vi "Lab Panel V4.86.vi"() -> ()   [LabVIEW 2013] (continued)
                    n882 = stacked-sequence {
                      seq-local: [w1543 _ _ _ _] -> [_ w1567 _ _ _]
                      tunnel: w1542 -> [w1548 _ _ _ _]
                      tunnel: w1541 -> [w1544 _ _ _ _]
                      tunnel: w1540 -> [w1558 _ _ _ _]
                      tunnel: w1539 -> [w1551 _ _ _ _]
                      tunnel: w1538 -> [w1546 _ _ _ _]
                      tunnel: [_ w1562 _ _ _] -> w1537
                      tunnel: w1536 -> [_ _ _ w1587 _]
                      tunnel: w1535 -> [_ _ _ w1586 _]
                      tunnel: w1534 -> [_ _ _ w1585 _]
                      frame #0 {
                        w1545 = "\\"
                        n883 = local read "SET LAB05-1"() -> (w1553:T5)
                        n884 = case shown="\"CYCLE TEST\"" w1558 {
                          tunnel: ["L05-1-CHART TEST-" "L05-1-CYCLE TEST-" "L05-1-T-RISE TEST-"] -> w1554
                          frame "CHART TEST", Default {
                          }
                          frame "CYCLE TEST" {
                          }
                          frame "T-RISE TEST" {
                          }
                        }
                        n885 = Unbundle(w1553) -> ("DESCRIPTION"=w1552:string)  [unwired: 4 out]
                        n886 = Concatenate Strings(w1548, "\\", w1546, w1545, w1544, w1545) -> (w1555:string)
                        n887 = String To Path(string=w1555) -> (path=w1557:path)
                        n888 = Concatenate Strings(w1555, w1554, w1552, "-", w1551, ".tdms") -> (w1543:string)
                        n889 = Create Folder(path (use dialog)=w1557) -> (error out=w1556:errorcluster)  [unwired: 2 in, 2 out]
                        n890 = global write "Global 1.vi" "LAB05-1 FILE"(w1543) -> ()
                        n891 = call <vilib>:"Clear Errors.vi"("error in (no error)"=w1556) -> ()  [unwired: 6 in, 1 out]
                      }
                      frame #1 {
                        (unwired) FALSE
                        n892 = String To Path(string=w1567) -> (path=w1563:path)
                        n893 = TDMS Open(6:FALSE, 10:T18."create or replace" ("operation (0:open)"), 11:w1563) -> (0:w1562:errorcluster, 3:→"TDMS LAB05-1":refnum<k34>)  [unwired: 4 in]
                      }
                      frame #2 {
                        n894 = local read "SET LAB05-1"() -> (w1573:T5)
                        n895 = local read "TDMS LAB05-1"() -> (w1584:refnum<k34>)
                        n896 = Build Array("Testers Name", "Description", "Set Test Cycles", "T-Rise minutes", "T-Rise Deg C") -> (w1574:string[])
                        n897 = Unbundle(w1573) -> ("NAME"=w1572:string, "DESCRIPTION"=w1571:string, "CYCLES"=w1570:dbl, "T-RISE mins"=w1569:dbl, "T-RISE deg C"=w1568:dbl)
                        n898 = Number To Decimal String(number=w1570) -> (decimal integer string=w1583:string)  [unwired: 1 in]
                        n899 = Number To Decimal String(number=w1569) -> (decimal integer string=w1582:string)  [unwired: 1 in]
                        n900 = Number To Decimal String(number=w1568) -> (decimal integer string=w1581:string)  [unwired: 1 in]
                        n901 = Build Array(w1572, w1571, w1583, w1582, w1581) -> (w1580:string[])
                        n902 = TDMS Set Properties(5:w1580, 7:w1574, 11:w1584) -> ()  [unwired: 3 in, 4 out]
                      }
                      frame #3 {
                        n903 = local read "DISP LAB05-1"() -> (w1589:T4)
                        n904 = Concatenate Strings("LAB05-1  ", w1587) -> (w1590:string)
                        n905 = Two Button Dialog(message=w1590, 1:w1585, 2:w1586) -> (T button?=w1592:bool)
                        n906 = case shown="True" w1592 {
                          tunnel: w1589 -> [w1599 w1600]
                          tunnel: [w1599 w1600] -> w1596
                          tunnel: [w1598 w1601] -> w1595
                          tunnel: [w1597 w1601] -> w1594
                          frame False {
                            n907 = Unbundle(w1599) -> ("CYCLE"=w1598:dbl, "MINS"=w1597:dbl)  [unwired: 1 out]
                          }
                          frame True {
                            w1601 = 0.0
                          }
                        }
                        n908 = Bundle(cluster=w1596, "CYCLE"=w1595, "MINS"=w1594, "STATUS"="RUN") -> (w1588:T4)
                        n909 = local write "DISP LAB05-1"(w1588) -> ()
                      }
                      frame #4 {
                        n910 = local read "SIG LAB05-1"() -> (w1604:T2)
                        n911 = local read "TEMP START LAB05-1"() -> (w1606:cluster{"TL":dbl, "TN":dbl})
                        n912 = Unbundle(w1604) -> ("Tmp Live"=w1603:dbl, "Tmp Neut"=w1602:dbl)  [unwired: 3 out]
                        n913 = Bundle(cluster=w1606, "TL"=w1603, "TN"=w1602) -> (w1605:cluster{"TL":dbl, "TN":dbl})
                        n914 = local write "TEMP START LAB05-1"(w1605) -> ()
                      }
                    }
                  }
                }
              }
              event "RUN LAB05-2": Value Change {
                n915 = event-data() -> ("NewVal"=w1610:bool)  [unwired: 1 in, 5 out]
                n916 = local write "run lab05-2"(w1610) -> ()
                n917 = case shown="True" w1610 {
                  tunnel: w1616 -> [_ w1652]
                  tunnel: w1615 -> [_ w1651]
                  tunnel: w1613 -> [w1618 w1650]
                  tunnel: w1614 -> [_ w1649]
                  tunnel: w1612 -> [_ w1648]
                  tunnel: [w1617 w1647] -> w1611
                  tunnel: w1609 -> [_ w1646]
                  tunnel: w1608 -> [_ w1645]
                  tunnel: w1607 -> [_ w1644]
                  frame False {
                    # "stop test"
                    n918 = stacked-sequence {
                      tunnel: w1618 -> [w1627 _]
                      tunnel: [w1619 _] -> w1617
                      frame #0 {
                        n919 = local read "DISP LAB05-2"() -> (w1626:T4)
                        n920 = Unbundle(w1626) -> ("CYCLE"=w1624:dbl, "MINS"=w1625:dbl)  [unwired: 1 out]
                        n921 = case shown="\"CYCLE TEST\"" w1627 {
                          tunnel: w1625 -> [_ _ w1634]
                          tunnel: w1624 -> [w1632 w1633 _]
                          tunnel: [w1632 w1633 w1634] -> w1623
                          frame "CHART TEST", Default {
                          }
                          frame "CYCLE TEST" {
                          }
                          frame "T-RISE TEST" {
                          }
                        }
                        n922 = local read "TDMS LAB05-2"() -> (w1631:refnum<k34>)
                        n923 = Build Array("STOPPED") -> (w1628:string[])
                        n924 = Build Array(w1623) -> (w1622:dbl[])
                        n925 = TDMS Write(0:w1631, 5:"TEST RESULT", 7:w1628, 9:w1622) -> (4:w1620:refnum<k34>, 15:w1621:errorcluster)  [unwired: 2 in, 2 out]
                        n926 = TDMS Close(8:w1621, 11:w1620) -> (0:w1619:errorcluster)  [unwired: 1 out]
                      }
                      frame #1 {
                        n927 = local read "DISP LAB05-2"() -> (w1638:T4)
                        n928 = stacked-sequence {
                          tunnel: "LAB05-2" -> [w1640 w1642]
                          frame #0 {
                            n929 = call "sub vi - defrag tdms v1.vi"("panel id"=w1640) -> ("error out"=w1639:errorcluster)  [unwired: 10 in]
                            n930 = local write "data file error"(w1639) -> ()
                          }
                          frame #1 {
                            n931 = local write "RESULT LAB05-2"(FALSE) -> ()
                            n932 = call "Save data file to network drive v2.vi"("panel id"=w1642) -> ("network file save error"=w1641:errorcluster)  [unwired: 9 in, 1 out]
                            n933 = local write "data file error"(w1641) -> ()
                          }
                        }
                        n934 = Bundle(cluster=w1638, "STATUS"="STOP") -> (w1636:T4)  [unwired: 2 in]
                        n935 = local write "DISP LAB05-2"(w1636) -> ()
                      }
                    }
                  }
                  frame True {
                    # "start new test and create test file"
                    n936 = stacked-sequence {
                      seq-local: [w1653 _ _ _ _] -> [_ w1677 _ _ _]
                      tunnel: w1652 -> [w1658 _ _ _ _]
                      tunnel: w1651 -> [w1654 _ _ _ _]
                      tunnel: w1650 -> [w1668 _ _ _ _]
                      tunnel: w1649 -> [w1661 _ _ _ _]
                      tunnel: w1648 -> [w1656 _ _ _ _]
                      tunnel: [_ w1672 _ _ _] -> w1647
                      tunnel: w1646 -> [_ _ _ w1697 _]
                      tunnel: w1645 -> [_ _ _ w1696 _]
                      tunnel: w1644 -> [_ _ _ w1695 _]
                      frame #0 {
                        w1655 = "\\"
                        n937 = local read "SET LAB05-2"() -> (w1663:T5)
                        n938 = case shown="\"CYCLE TEST\"" w1668 {
                          tunnel: ["L05-2-CHART TEST-" "L05-2-CYCLE TEST-" "L05-2-T-RISE TEST-"] -> w1664
                          frame "CHART TEST", Default {
                          }
                          frame "CYCLE TEST" {
                          }
                          frame "T-RISE TEST" {
                          }
                        }
                        n939 = Unbundle(w1663) -> ("DESCRIPTION"=w1662:string)  [unwired: 4 out]
                        n940 = Concatenate Strings(w1658, "\\", w1656, w1655, w1654, w1655) -> (w1665:string)
                        n941 = String To Path(string=w1665) -> (path=w1667:path)
                        n942 = Concatenate Strings(w1665, w1664, w1662, "-", w1661, ".tdms") -> (w1653:string)
                        n943 = Create Folder(path (use dialog)=w1667) -> (error out=w1666:errorcluster)  [unwired: 2 in, 2 out]
                        n944 = global write "Global 1.vi" "LAB05-2 FILE"(w1653) -> ()
                        n945 = call <vilib>:"Clear Errors.vi"("error in (no error)"=w1666) -> ()  [unwired: 6 in, 1 out]
                      }
                      frame #1 {
                        (unwired) FALSE
                        n946 = String To Path(string=w1677) -> (path=w1673:path)
                        n947 = TDMS Open(6:FALSE, 10:T18."create or replace" ("operation (0:open)"), 11:w1673) -> (0:w1672:errorcluster, 3:→"TDMS LAB05-2":refnum<k34>)  [unwired: 4 in]
                      }
                      frame #2 {
                        n948 = local read "SET LAB05-2"() -> (w1683:T5)
                        n949 = local read "TDMS LAB05-2"() -> (w1694:refnum<k34>)
                        n950 = Build Array("Testers Name", "Description", "Set Test Cycles", "T-Rise minutes", "T-Rise Deg C") -> (w1684:string[])
                        n951 = Unbundle(w1683) -> ("NAME"=w1682:string, "DESCRIPTION"=w1681:string, "CYCLES"=w1680:dbl, "T-RISE mins"=w1679:dbl, "T-RISE deg C"=w1678:dbl)
                        n952 = Number To Decimal String(number=w1680) -> (decimal integer string=w1693:string)  [unwired: 1 in]
                        n953 = Number To Decimal String(number=w1679) -> (decimal integer string=w1692:string)  [unwired: 1 in]
                        n954 = Number To Decimal String(number=w1678) -> (decimal integer string=w1691:string)  [unwired: 1 in]
                        n955 = Build Array(w1682, w1681, w1693, w1692, w1691) -> (w1690:string[])
                        n956 = TDMS Set Properties(5:w1690, 7:w1684, 11:w1694) -> ()  [unwired: 3 in, 4 out]
                      }
                      frame #3 {
                        n957 = local read "DISP LAB05-2"() -> (w1699:T4)
                        n958 = Concatenate Strings("LAB05-2  ", w1697) -> (w1700:string)
                        n959 = Two Button Dialog(message=w1700, 1:w1695, 2:w1696) -> (T button?=w1702:bool)
                        n960 = case shown="True" w1702 {
                          tunnel: w1699 -> [w1709 w1710]
                          tunnel: [w1709 w1710] -> w1706
                          tunnel: [w1708 w1711] -> w1705
                          tunnel: [w1707 w1711] -> w1704
                          frame False {
                            n961 = Unbundle(w1709) -> ("CYCLE"=w1708:dbl, "MINS"=w1707:dbl)  [unwired: 1 out]
                          }
                          frame True {
                            w1711 = 0.0
                          }
                        }
                        n962 = Bundle(cluster=w1706, "CYCLE"=w1705, "MINS"=w1704, "STATUS"="RUN") -> (w1698:T4)
                        n963 = local write "DISP LAB05-2"(w1698) -> ()
                      }
                      frame #4 {
                        n964 = local read "SIG LAB05-2"() -> (w1714:T2)
                        n965 = local read "TEMP START LAB05-2"() -> (w1716:cluster{"TL":dbl, "TN":dbl})
                        n966 = Unbundle(w1714) -> ("Tmp Live"=w1713:dbl, "Tmp Neut"=w1712:dbl)  [unwired: 3 out]
                        n967 = Bundle(cluster=w1716, "TL"=w1713, "TN"=w1712) -> (w1715:cluster{"TL":dbl, "TN":dbl})
                        n968 = local write "TEMP START LAB05-2"(w1715) -> ()
                      }
                    }
                  }
                }
              }
            }
            n969 = local write "data file error"(w588) -> ()
          }
          frame #4 {
            # "check if test cycles reached for cycle tests, if so then test pass"
            n970 = stacked-sequence {
              tunnel: w1736 -> [_ _ _ _ _ _ _ _ _ _]
              tunnel: w1735 -> [_ _ _ _ _ _ _ _ _ _]
              tunnel: w1734 -> [_ _ _ _ _ _ _ _ _ _]
              tunnel: w1733 -> [_ _ _ _ _ _ _ _ _ _]
              tunnel: w1732 -> [_ _ _ _ _ _ _ _ _ _]
              tunnel: w1731 -> [_ _ _ _ _ _ _ _ _ _]
              tunnel: w1730 -> [_ _ _ _ _ _ _ _ _ _]
              tunnel: w1729 -> [_ _ _ _ _ _ _ _ _ _]
              tunnel: w1728 -> [_ _ _ _ _ _ _ _ _ _]
              tunnel: w1727 -> [_ _ _ _ _ _ _ _ _ _]
              tunnel: w1726 -> [w1742 _ _ _ _ _ _ _ _ _]
              tunnel: w1725 -> [_ w1777 _ _ _ _ _ _ _ _]
              tunnel: w1724 -> [_ _ w1817 _ _ _ _ _ _ _]
              tunnel: w1723 -> [_ _ _ w1857 _ _ _ _ _ _]
              tunnel: w1722 -> [_ _ _ _ w1897 _ _ _ _ _]
              tunnel: w1721 -> [_ _ _ _ _ w1937 _ _ _ _]
              tunnel: w1720 -> [_ _ _ _ _ _ w1977 _ _ _]
              tunnel: w1719 -> [_ _ _ _ _ _ _ w2017 _ _]
              tunnel: w1718 -> [_ _ _ _ _ _ _ _ w2057 _]
              tunnel: w1717 -> [_ _ _ _ _ _ _ _ _ w2097]
              frame #0 {
                # "LAB01-1"
                n971 = Less?(x=w1742, y=2) -> (x < y?=w1740:bool)
                n972 = local read "DISP LAB01-1"() -> (w1743:T4)
                n973 = Unbundle(w1743) -> ("STATUS"=w1737:string)  [unwired: 2 out]
                n974 = Equal?(x=w1737, y="RUN") -> (x = y?=w1739:bool)
                n975 = And(x=w1739, y=w1740) -> (x .and. y?=w1738:bool)
                n976 = case shown="True" w1738 {
                  tunnel: w1743 -> [_ w1748]
                  tunnel: w1742 -> [_ w1752]
                  frame False {
                  }
                  frame True {
                    n977 = local read "SET LAB01-1"() -> (w1754:T5)
                    n978 = local read "TDMS LAB01-1"() -> (w1747:refnum<k34>)
                    n979 = Unbundle(w1754) -> ("CYCLES"=w1745:dbl, "T-RISE mins"=w1751:dbl)  [unwired: 3 out]
                    n980 = case shown="\"CYCLE TEST\"" w1752 {
                      tunnel: w1751 -> [_ _ w1761]
                      tunnel: [w1756 w1758 w1761] -> w1750
                      tunnel: w1745 -> [w1756 w1758 _]
                      tunnel: ["CHART PASS" "CYCLE PASS" "T-RISE PASS"] -> w1749
                      frame "CHART TEST", Default {
                      }
                      frame "CYCLE TEST" {
                      }
                      frame "T-RISE TEST" {
                      }
                    }
                    n981 = Unbundle(w1748) -> ("CYCLE"=w1753:dbl)  [unwired: 2 out]
                    n982 = Increment(x=w1745) -> (x+1=w1746:dbl)
                    n983 = Greater Or Equal?(x=w1753, y=w1746) -> (x >= y?=w1755:bool)
                    n984 = case shown="True" w1755 {
                      tunnel: w1750 -> [w1765 _]
                      tunnel: w1749 -> [w1764 _]
                      tunnel: w1748 -> [w1763 _]
                      tunnel: w1747 -> [w1762 _]
                      frame True {
                        n985 = stacked-sequence {
                          tunnel: w1765 -> [w1769 _]
                          tunnel: w1764 -> [w1767 w1773]
                          tunnel: w1763 -> [_ w1776]
                          tunnel: w1762 -> [w1766 _]
                          frame #0 {
                            n986 = Build Array(w1767) -> (w1770:string[])
                            n987 = Build Array(w1769) -> (w1768:dbl[])
                            n988 = TDMS Write(0:w1766, 5:"TEST PASS", 7:w1770, 9:w1768) -> (15:w1772:errorcluster)  [unwired: 2 in, 3 out]
                            n989 = local write "data file error"(w1772) -> ()
                          }
                          frame #1 {
                            n990 = Bundle(cluster=w1776, "STATUS"=w1773) -> (w1774:T4)  [unwired: 2 in]
                            n991 = local write "RESULT LAB01-1"(TRUE) -> ()
                            n992 = local write "DISP LAB01-1"(w1774) -> ()
                          }
                        }
                      }
                      frame False {
                      }
                    }
                  }
                }
              }
              frame #1 {
                # "LAB01-2"
                n993 = Less?(x=w1777, y=2) -> (x < y?=w1780:bool)
                n994 = local read "DISP LAB01-2"() -> (w1782:T4)
                n995 = Unbundle(w1782) -> ("STATUS"=w1783:string)  [unwired: 2 out]
                n996 = Equal?(x=w1783, y="RUN") -> (x = y?=w1779:bool)
                n997 = And(x=w1779, y=w1780) -> (x .and. y?=w1778:bool)
                n998 = case shown="True" w1778 {
                  tunnel: w1782 -> [_ w1788]
                  tunnel: w1777 -> [_ w1792]
                  frame False {
                  }
                  frame True {
                    n999 = local read "SET LAB01-2"() -> (w1794:T5)
                    n1000 = local read "TDMS LAB01-2"() -> (w1787:refnum<k34>)
                    n1001 = Unbundle(w1794) -> ("CYCLES"=w1785:dbl, "T-RISE mins"=w1791:dbl)  [unwired: 3 out]
                    n1002 = case shown="\"T-RISE TEST\"" w1792 {
                      tunnel: w1791 -> [_ _ w1801]
                      tunnel: [w1796 w1798 w1801] -> w1790
                      tunnel: w1785 -> [w1796 w1798 _]
                      tunnel: ["CHART PASS" "CYCLE PASS" "T-RISE PASS"] -> w1789
                      frame "CHART TEST", Default {
                      }
                      frame "CYCLE TEST" {
                      }
                      frame "T-RISE TEST" {
                      }
                    }
                    n1003 = Unbundle(w1788) -> ("CYCLE"=w1793:dbl)  [unwired: 2 out]
                    n1004 = Increment(x=w1785) -> (x+1=w1786:dbl)
                    n1005 = Greater Or Equal?(x=w1793, y=w1786) -> (x >= y?=w1795:bool)
                    n1006 = case shown="True" w1795 {
                      tunnel: w1790 -> [w1805 _]
                      tunnel: w1789 -> [w1804 _]
                      tunnel: w1788 -> [w1803 _]
                      tunnel: w1787 -> [w1802 _]
                      frame True {
                        n1007 = stacked-sequence {
                          tunnel: w1805 -> [w1809 _]
                          tunnel: w1804 -> [w1807 w1813]
                          tunnel: w1803 -> [_ w1816]
                          tunnel: w1802 -> [w1806 _]
                          frame #0 {
                            n1008 = Build Array(w1807) -> (w1810:string[])
                            n1009 = Build Array(w1809) -> (w1808:dbl[])
                            n1010 = TDMS Write(0:w1806, 5:"TEST PASS", 7:w1810, 9:w1808) -> (15:w1812:errorcluster)  [unwired: 2 in, 3 out]
                            n1011 = local write "data file error"(w1812) -> ()
                          }
                          frame #1 {
                            n1012 = Bundle(cluster=w1816, "STATUS"=w1813) -> (w1814:T4)  [unwired: 2 in]
                            n1013 = local write "RESULT LAB01-2"(TRUE) -> ()
                            n1014 = local write "DISP LAB01-2"(w1814) -> ()
                          }
                        }
                      }
                      frame False {
                      }
                    }
                  }
                }
              }
              frame #2 {
                # "LAB02-1"
                n1015 = Less?(x=w1817, y=2) -> (x < y?=w1820:bool)
                n1016 = local read "DISP LAB02-1"() -> (w1822:T4)
                n1017 = Unbundle(w1822) -> ("STATUS"=w1823:string)  [unwired: 2 out]
                n1018 = Equal?(x=w1823, y="RUN") -> (x = y?=w1819:bool)
                n1019 = And(x=w1819, y=w1820) -> (x .and. y?=w1818:bool)
                n1020 = case shown="True" w1818 {
                  tunnel: w1822 -> [_ w1828]
                  tunnel: w1817 -> [_ w1832]
                  frame False {
                  }
                  frame True {
                    n1021 = local read "SET LAB02-1"() -> (w1834:T5)
                    n1022 = local read "TDMS LAB02-1"() -> (w1827:refnum<k34>)
                    n1023 = Unbundle(w1828) -> ("CYCLE"=w1833:dbl)  [unwired: 2 out]
                    n1024 = Unbundle(w1834) -> ("CYCLES"=w1825:dbl, "T-RISE mins"=w1831:dbl)  [unwired: 3 out]
                    n1025 = case shown="\"T-RISE TEST\"" w1832 {
                      tunnel: w1831 -> [_ _ w1841]
                      tunnel: [w1836 w1838 w1841] -> w1830
                      tunnel: w1825 -> [w1836 w1838 _]
                      tunnel: ["CHART PASS" "CYCLE PASS" "T-RISE PASS"] -> w1829
                      frame "CHART TEST", Default {
                      }
                      frame "CYCLE TEST" {
                      }
                      frame "T-RISE TEST" {
                      }
                    }
                    n1026 = Increment(x=w1825) -> (x+1=w1826:dbl)
                    n1027 = Greater Or Equal?(x=w1833, y=w1826) -> (x >= y?=w1835:bool)
                    n1028 = case shown="True" w1835 {
                      tunnel: w1830 -> [w1845 _]
                      tunnel: w1829 -> [w1844 _]
                      tunnel: w1828 -> [w1843 _]
                      tunnel: w1827 -> [w1842 _]
                      frame True {
                        n1029 = stacked-sequence {
                          tunnel: w1845 -> [w1849 _]
                          tunnel: w1844 -> [w1847 w1853]
                          tunnel: w1843 -> [_ w1856]
                          tunnel: w1842 -> [w1846 _]
                          frame #0 {
                            n1030 = Build Array(w1847) -> (w1850:string[])
                            n1031 = Build Array(w1849) -> (w1848:dbl[])
                            n1032 = TDMS Write(0:w1846, 5:"TEST PASS", 7:w1850, 9:w1848) -> (15:w1852:errorcluster)  [unwired: 2 in, 3 out]
                            n1033 = local write "data file error"(w1852) -> ()
                          }
                          frame #1 {
                            n1034 = Bundle(cluster=w1856, "STATUS"=w1853) -> (w1854:T4)  [unwired: 2 in]
                            n1035 = local write "RESULT LAB02-1"(TRUE) -> ()
                            n1036 = local write "DISP LAB02-1"(w1854) -> ()
                          }
                        }
                      }
                      frame False {
                      }
                    }
                  }
                }
              }
              frame #3 {
                # "LAB02-2"
                n1037 = Less?(x=w1857, y=2) -> (x < y?=w1860:bool)
                n1038 = local read "DISP LAB02-2"() -> (w1862:T4)
                n1039 = Unbundle(w1862) -> ("STATUS"=w1863:string)  [unwired: 2 out]
                n1040 = Equal?(x=w1863, y="RUN") -> (x = y?=w1859:bool)
                n1041 = And(x=w1859, y=w1860) -> (x .and. y?=w1858:bool)
                n1042 = case shown="True" w1858 {
                  tunnel: w1862 -> [_ w1868]
                  tunnel: w1857 -> [_ w1872]
                  frame False {
                  }
                  frame True {
                    n1043 = local read "SET LAB02-2"() -> (w1874:T5)
                    n1044 = local read "TDMS LAB02-2"() -> (w1867:refnum<k34>)
                    n1045 = Unbundle(w1868) -> ("CYCLE"=w1873:dbl)  [unwired: 2 out]
                    n1046 = Unbundle(w1874) -> ("CYCLES"=w1865:dbl, "T-RISE mins"=w1871:dbl)  [unwired: 3 out]
                    n1047 = case shown="\"T-RISE TEST\"" w1872 {
                      tunnel: w1871 -> [_ _ w1881]
                      tunnel: [w1876 w1878 w1881] -> w1870
                      tunnel: w1865 -> [w1876 w1878 _]
                      tunnel: ["CHART PASS" "CYCLE PASS" "T-RISE PASS"] -> w1869
                      frame "CHART TEST", Default {
                      }
                      frame "CYCLE TEST" {
                      }
                      frame "T-RISE TEST" {
                      }
                    }
                    n1048 = Increment(x=w1865) -> (x+1=w1866:dbl)
                    n1049 = Greater Or Equal?(x=w1873, y=w1866) -> (x >= y?=w1875:bool)
                    n1050 = case shown="True" w1875 {
                      tunnel: w1870 -> [w1885 _]
                      tunnel: w1869 -> [w1884 _]
                      tunnel: w1868 -> [w1883 _]
                      tunnel: w1867 -> [w1882 _]
                      frame True {
                        n1051 = stacked-sequence {
                          tunnel: w1885 -> [w1889 _]
                          tunnel: w1884 -> [w1887 w1893]
                          tunnel: w1883 -> [_ w1896]
                          tunnel: w1882 -> [w1886 _]
                          frame #0 {
                            n1052 = Build Array(w1887) -> (w1890:string[])
                            n1053 = Build Array(w1889) -> (w1888:dbl[])
                            n1054 = TDMS Write(0:w1886, 5:"TEST PASS", 7:w1890, 9:w1888) -> (15:w1892:errorcluster)  [unwired: 2 in, 3 out]
                            n1055 = local write "data file error"(w1892) -> ()
                          }
                          frame #1 {
                            n1056 = Bundle(cluster=w1896, "STATUS"=w1893) -> (w1894:T4)  [unwired: 2 in]
                            n1057 = local write "RESULT LAB02-2"(TRUE) -> ()
                            n1058 = local write "DISP LAB02-2"(w1894) -> ()
                          }
                        }
                      }
                      frame False {
                      }
                    }
                  }
                }
              }
              frame #4 {
                # "LAB03-1"
                n1059 = Less?(x=w1897, y=2) -> (x < y?=w1900:bool)
                n1060 = local read "DISP LAB03-1"() -> (w1902:T4)
                n1061 = Unbundle(w1902) -> ("STATUS"=w1903:string)  [unwired: 2 out]
                n1062 = Equal?(x=w1903, y="RUN") -> (x = y?=w1899:bool)
                n1063 = And(x=w1899, y=w1900) -> (x .and. y?=w1898:bool)
                n1064 = case shown="True" w1898 {
                  tunnel: w1902 -> [_ w1908]
                  tunnel: w1897 -> [_ w1912]
                  frame False {
                  }
                  frame True {
                    n1065 = local read "SET LAB03-1"() -> (w1914:T5)
                    n1066 = local read "TDMS LAB03-1"() -> (w1907:refnum<k34>)
                    n1067 = Unbundle(w1908) -> ("CYCLE"=w1913:dbl)  [unwired: 2 out]
                    n1068 = Unbundle(w1914) -> ("CYCLES"=w1905:dbl, "T-RISE mins"=w1911:dbl)  [unwired: 3 out]
                    n1069 = case shown="\"T-RISE TEST\"" w1912 {
                      tunnel: w1911 -> [_ _ w1921]
                      tunnel: [w1916 w1918 w1921] -> w1910
                      tunnel: w1905 -> [w1916 w1918 _]
                      tunnel: ["CHART PASS" "CYCLE PASS" "T-RISE PASS"] -> w1909
                      frame "CHART TEST", Default {
                      }
                      frame "CYCLE TEST" {
                      }
                      frame "T-RISE TEST" {
                      }
                    }
                    n1070 = Increment(x=w1905) -> (x+1=w1906:dbl)
                    n1071 = Greater Or Equal?(x=w1913, y=w1906) -> (x >= y?=w1915:bool)
                    n1072 = case shown="True" w1915 {
                      tunnel: w1910 -> [w1925 _]
                      tunnel: w1909 -> [w1924 _]
                      tunnel: w1908 -> [w1923 _]
                      tunnel: w1907 -> [w1922 _]
                      frame True {
                        n1073 = stacked-sequence {
                          tunnel: w1925 -> [w1929 _]
                          tunnel: w1924 -> [w1927 w1933]
                          tunnel: w1923 -> [_ w1936]
                          tunnel: w1922 -> [w1926 _]
                          frame #0 {
                            n1074 = Build Array(w1927) -> (w1930:string[])
                            n1075 = Build Array(w1929) -> (w1928:dbl[])
                            n1076 = TDMS Write(0:w1926, 5:"TEST PASS", 7:w1930, 9:w1928) -> (15:w1932:errorcluster)  [unwired: 2 in, 3 out]
                            n1077 = local write "data file error"(w1932) -> ()
                          }
                          frame #1 {
                            n1078 = Bundle(cluster=w1936, "STATUS"=w1933) -> (w1934:T4)  [unwired: 2 in]
                            n1079 = local write "RESULT LAB03-1"(TRUE) -> ()
                            n1080 = local write "DISP LAB03-1"(w1934) -> ()
                          }
                        }
                      }
                      frame False {
                      }
                    }
                  }
                }
              }
              frame #5 {
                # "LAB03-2"
                n1081 = Less?(x=w1937, y=2) -> (x < y?=w1940:bool)
                n1082 = local read "DISP LAB03-2"() -> (w1942:T4)
                n1083 = Unbundle(w1942) -> ("STATUS"=w1943:string)  [unwired: 2 out]
                n1084 = Equal?(x=w1943, y="RUN") -> (x = y?=w1939:bool)
                n1085 = And(x=w1939, y=w1940) -> (x .and. y?=w1938:bool)
                n1086 = case shown="True" w1938 {
                  tunnel: w1942 -> [_ w1948]
                  tunnel: w1937 -> [_ w1952]
                  frame False {
                  }
                  frame True {
                    n1087 = local read "SET LAB03-2"() -> (w1954:T5)
                    n1088 = local read "TDMS LAB03-2"() -> (w1947:refnum<k34>)
                    n1089 = Unbundle(w1948) -> ("CYCLE"=w1953:dbl)  [unwired: 2 out]
                    n1090 = Unbundle(w1954) -> ("CYCLES"=w1945:dbl, "T-RISE mins"=w1951:dbl)  [unwired: 3 out]
                    n1091 = case shown="\"T-RISE TEST\"" w1952 {
                      tunnel: w1951 -> [_ _ w1961]
                      tunnel: [w1956 w1958 w1961] -> w1950
                      tunnel: w1945 -> [w1956 w1958 _]
                      tunnel: ["CHART PASS" "CYCLE PASS" "T-RISE PASS"] -> w1949
                      frame "CHART TEST", Default {
                      }
                      frame "CYCLE TEST" {
                      }
                      frame "T-RISE TEST" {
                      }
                    }
                    n1092 = Increment(x=w1945) -> (x+1=w1946:dbl)
                    n1093 = Greater Or Equal?(x=w1953, y=w1946) -> (x >= y?=w1955:bool)
                    n1094 = case shown="True" w1955 {
                      tunnel: w1950 -> [w1965 _]
                      tunnel: w1949 -> [w1964 _]
                      tunnel: w1948 -> [w1963 _]
                      tunnel: w1947 -> [w1962 _]
                      frame True {
                        n1095 = stacked-sequence {
                          tunnel: w1965 -> [w1969 _]
                          tunnel: w1964 -> [w1967 w1973]
                          tunnel: w1963 -> [_ w1976]
                          tunnel: w1962 -> [w1966 _]
                          frame #0 {
                            n1096 = Build Array(w1967) -> (w1970:string[])
                            n1097 = Build Array(w1969) -> (w1968:dbl[])
                            n1098 = TDMS Write(0:w1966, 5:"TEST PASS", 7:w1970, 9:w1968) -> (15:w1972:errorcluster)  [unwired: 2 in, 3 out]
                            n1099 = local write "data file error"(w1972) -> ()
                          }
                          frame #1 {
                            n1100 = Bundle(cluster=w1976, "STATUS"=w1973) -> (w1974:T4)  [unwired: 2 in]
                            n1101 = local write "RESULT LAB03-2"(TRUE) -> ()
                            n1102 = local write "DISP LAB03-2"(w1974) -> ()
                          }
                        }
                      }
                      frame False {
                      }
                    }
                  }
                }
              }
              frame #6 {
                # "LAB04-1"
                n1103 = Less?(x=w1977, y=2) -> (x < y?=w1980:bool)
                n1104 = local read "DISP LAB04-1"() -> (w1982:T4)
                n1105 = Unbundle(w1982) -> ("STATUS"=w1983:string)  [unwired: 2 out]
                n1106 = Equal?(x=w1983, y="RUN") -> (x = y?=w1979:bool)
                n1107 = And(x=w1979, y=w1980) -> (x .and. y?=w1978:bool)
                n1108 = case shown="True" w1978 {
                  tunnel: w1982 -> [_ w1988]
                  tunnel: w1977 -> [_ w1992]
                  frame False {
                  }
                  frame True {
                    n1109 = local read "SET LAB04-1"() -> (w1994:T5)
                    n1110 = local read "TDMS LAB04-1"() -> (w1987:refnum<k34>)
                    n1111 = Unbundle(w1988) -> ("CYCLE"=w1993:dbl)  [unwired: 2 out]
                    n1112 = Unbundle(w1994) -> ("CYCLES"=w1985:dbl, "T-RISE mins"=w1991:dbl)  [unwired: 3 out]
                    n1113 = case shown="\"T-RISE TEST\"" w1992 {
                      tunnel: w1991 -> [_ _ w2001]
                      tunnel: [w1996 w1998 w2001] -> w1990
                      tunnel: w1985 -> [w1996 w1998 _]
                      tunnel: ["CHART PASS" "CYCLE PASS" "T-RISE PASS"] -> w1989
                      frame "CHART TEST", Default {
                      }
                      frame "CYCLE TEST" {
                      }
                      frame "T-RISE TEST" {
                      }
                    }
                    n1114 = Increment(x=w1985) -> (x+1=w1986:dbl)
                    n1115 = Greater Or Equal?(x=w1993, y=w1986) -> (x >= y?=w1995:bool)
                    n1116 = case shown="True" w1995 {
                      tunnel: w1990 -> [w2005 _]
                      tunnel: w1989 -> [w2004 _]
                      tunnel: w1988 -> [w2003 _]
                      tunnel: w1987 -> [w2002 _]
                      frame True {
                        n1117 = stacked-sequence {
                          tunnel: w2005 -> [w2009 _]
                          tunnel: w2004 -> [w2007 w2013]
                          tunnel: w2003 -> [_ w2016]
                          tunnel: w2002 -> [w2006 _]
                          frame #0 {
                            n1118 = Build Array(w2007) -> (w2010:string[])
                            n1119 = Build Array(w2009) -> (w2008:dbl[])
                            n1120 = TDMS Write(0:w2006, 5:"TEST PASS", 7:w2010, 9:w2008) -> (15:w2012:errorcluster)  [unwired: 2 in, 3 out]
                            n1121 = local write "data file error"(w2012) -> ()
                          }
                          frame #1 {
                            n1122 = Bundle(cluster=w2016, "STATUS"=w2013) -> (w2014:T4)  [unwired: 2 in]
                            n1123 = local write "RESULT LAB04-1"(TRUE) -> ()
                            n1124 = local write "DISP LAB04-1"(w2014) -> ()
                          }
                        }
                      }
                      frame False {
                      }
                    }
                  }
                }
              }
              frame #7 {
                # "LAB04-2"
                n1125 = Less?(x=w2017, y=2) -> (x < y?=w2020:bool)
                n1126 = local read "DISP LAB04-2"() -> (w2022:T4)
                n1127 = Unbundle(w2022) -> ("STATUS"=w2023:string)  [unwired: 2 out]
                n1128 = Equal?(x=w2023, y="RUN") -> (x = y?=w2019:bool)
                n1129 = And(x=w2019, y=w2020) -> (x .and. y?=w2018:bool)
                n1130 = case shown="True" w2018 {
                  tunnel: w2022 -> [_ w2028]
                  tunnel: w2017 -> [_ w2032]
                  frame False {
                  }
                  frame True {
                    n1131 = local read "SET LAB04-2"() -> (w2034:T5)
                    n1132 = local read "TDMS LAB04-2"() -> (w2027:refnum<k34>)
                    n1133 = Unbundle(w2028) -> ("CYCLE"=w2033:dbl)  [unwired: 2 out]
                    n1134 = Unbundle(w2034) -> ("CYCLES"=w2025:dbl, "T-RISE mins"=w2031:dbl)  [unwired: 3 out]
                    n1135 = case shown="\"T-RISE TEST\"" w2032 {
                      tunnel: w2031 -> [_ _ w2041]
                      tunnel: [w2036 w2038 w2041] -> w2030
                      tunnel: w2025 -> [w2036 w2038 _]
                      tunnel: ["CHART PASS" "CYCLE PASS" "T-RISE PASS"] -> w2029
                      frame "CHART TEST", Default {
                      }
                      frame "CYCLE TEST" {
                      }
                      frame "T-RISE TEST" {
                      }
                    }
                    n1136 = Increment(x=w2025) -> (x+1=w2026:dbl)
                    n1137 = Greater Or Equal?(x=w2033, y=w2026) -> (x >= y?=w2035:bool)
                    n1138 = case shown="True" w2035 {
                      tunnel: w2030 -> [w2045 _]
                      tunnel: w2029 -> [w2044 _]
                      tunnel: w2028 -> [w2043 _]
                      tunnel: w2027 -> [w2042 _]
                      frame True {
                        n1139 = stacked-sequence {
                          tunnel: w2045 -> [w2049 _]
                          tunnel: w2044 -> [w2047 w2053]
                          tunnel: w2043 -> [_ w2056]
                          tunnel: w2042 -> [w2046 _]
                          frame #0 {
                            n1140 = Build Array(w2047) -> (w2050:string[])
                            n1141 = Build Array(w2049) -> (w2048:dbl[])
                            n1142 = TDMS Write(0:w2046, 5:"TEST PASS", 7:w2050, 9:w2048) -> (15:w2052:errorcluster)  [unwired: 2 in, 3 out]
                            n1143 = local write "data file error"(w2052) -> ()
                          }
                          frame #1 {
                            n1144 = Bundle(cluster=w2056, "STATUS"=w2053) -> (w2054:T4)  [unwired: 2 in]
                            n1145 = local write "RESULT LAB04-2"(TRUE) -> ()
                            n1146 = local write "DISP LAB04-2"(w2054) -> ()
                          }
                        }
                      }
                      frame False {
                      }
                    }
                  }
                }
              }
              frame #8 {
                # "LAB05-1"
                n1147 = Less?(x=w2057, y=2) -> (x < y?=w2060:bool)
                n1148 = local read "DISP LAB05-1"() -> (w2062:T4)
                n1149 = Unbundle(w2062) -> ("STATUS"=w2063:string)  [unwired: 2 out]
                n1150 = Equal?(x=w2063, y="RUN") -> (x = y?=w2059:bool)
                n1151 = And(x=w2059, y=w2060) -> (x .and. y?=w2058:bool)
                n1152 = case shown="True" w2058 {
                  tunnel: w2062 -> [_ w2068]
                  tunnel: w2057 -> [_ w2072]
                  frame False {
                  }
                  frame True {
                    n1153 = local read "SET LAB05-1"() -> (w2074:T5)
                    n1154 = local read "TDMS LAB05-1"() -> (w2067:refnum<k34>)
                    n1155 = Unbundle(w2068) -> ("CYCLE"=w2073:dbl)  [unwired: 2 out]
                    n1156 = Unbundle(w2074) -> ("CYCLES"=w2065:dbl, "T-RISE mins"=w2071:dbl)  [unwired: 3 out]
                    n1157 = case shown="\"T-RISE TEST\"" w2072 {
                      tunnel: w2071 -> [_ _ w2081]
                      tunnel: [w2076 w2078 w2081] -> w2070
                      tunnel: w2065 -> [w2076 w2078 _]
                      tunnel: ["CHART PASS" "CYCLE PASS" "T-RISE PASS"] -> w2069
                      frame "CHART TEST", Default {
                      }
                      frame "CYCLE TEST" {
                      }
                      frame "T-RISE TEST" {
                      }
                    }
                    n1158 = Increment(x=w2065) -> (x+1=w2066:dbl)
                    n1159 = Greater Or Equal?(x=w2073, y=w2066) -> (x >= y?=w2075:bool)
                    n1160 = case shown="True" w2075 {
                      tunnel: w2070 -> [w2085 _]
                      tunnel: w2069 -> [w2084 _]
                      tunnel: w2068 -> [w2083 _]
                      tunnel: w2067 -> [w2082 _]
                      frame True {
                        n1161 = stacked-sequence {
                          tunnel: w2085 -> [w2089 _]
                          tunnel: w2084 -> [w2087 w2093]
                          tunnel: w2083 -> [_ w2096]
                          tunnel: w2082 -> [w2086 _]
                          frame #0 {
                            n1162 = Build Array(w2087) -> (w2090:string[])
                            n1163 = Build Array(w2089) -> (w2088:dbl[])
                            n1164 = TDMS Write(0:w2086, 5:"TEST PASS", 7:w2090, 9:w2088) -> (15:w2092:errorcluster)  [unwired: 2 in, 3 out]
                            n1165 = local write "data file error"(w2092) -> ()
                          }
                          frame #1 {
                            n1166 = Bundle(cluster=w2096, "STATUS"=w2093) -> (w2094:T4)  [unwired: 2 in]
                            n1167 = local write "RESULT LAB05-1"(TRUE) -> ()
                            n1168 = local write "DISP LAB05-1"(w2094) -> ()
                          }
                        }
                      }
                      frame False {
                      }
                    }
                  }
                }
              }
              frame #9 {
                # "LAB05-2"
                n1169 = Less?(x=w2097, y=2) -> (x < y?=w2100:bool)
                n1170 = local read "DISP LAB05-2"() -> (w2102:T4)
                n1171 = Unbundle(w2102) -> ("STATUS"=w2103:string)  [unwired: 2 out]
                n1172 = Equal?(x=w2103, y="RUN") -> (x = y?=w2099:bool)
                n1173 = And(x=w2099, y=w2100) -> (x .and. y?=w2098:bool)
                n1174 = case shown="True" w2098 {
                  tunnel: w2102 -> [_ w2108]
                  tunnel: w2097 -> [_ w2112]
                  frame False {
                  }
                  frame True {
                    n1175 = local read "SET LAB05-2"() -> (w2114:T5)
                    n1176 = local read "TDMS LAB05-2"() -> (w2107:refnum<k34>)
                    n1177 = Unbundle(w2108) -> ("CYCLE"=w2113:dbl)  [unwired: 2 out]
                    n1178 = Unbundle(w2114) -> ("CYCLES"=w2105:dbl, "T-RISE mins"=w2111:dbl)  [unwired: 3 out]
                    n1179 = case shown="\"T-RISE TEST\"" w2112 {
                      tunnel: w2111 -> [_ _ w2121]
                      tunnel: [w2116 w2118 w2121] -> w2110
                      tunnel: w2105 -> [w2116 w2118 _]
                      tunnel: ["CHART PASS" "CYCLE PASS" "T-RISE PASS"] -> w2109
                      frame "CHART TEST", Default {
                      }
                      frame "CYCLE TEST" {
                      }
                      frame "T-RISE TEST" {
                      }
                    }
                    n1180 = Increment(x=w2105) -> (x+1=w2106:dbl)
                    n1181 = Greater Or Equal?(x=w2113, y=w2106) -> (x >= y?=w2115:bool)
                    n1182 = case shown="True" w2115 {
                      tunnel: w2110 -> [w2125 _]
                      tunnel: w2109 -> [w2124 _]
                      tunnel: w2108 -> [w2123 _]
                      tunnel: w2107 -> [w2122 _]
                      frame True {
                        n1183 = stacked-sequence {
                          tunnel: w2125 -> [w2129 _]
                          tunnel: w2124 -> [w2127 w2133]
                          tunnel: w2123 -> [_ w2136]
                          tunnel: w2122 -> [w2126 _]
                          frame #0 {
                            n1184 = Build Array(w2127) -> (w2130:string[])
                            n1185 = Build Array(w2129) -> (w2128:dbl[])
                            n1186 = TDMS Write(0:w2126, 5:"TEST PASS", 7:w2130, 9:w2128) -> (15:w2132:errorcluster)  [unwired: 2 in, 3 out]
                            n1187 = local write "data file error"(w2132) -> ()
                          }
                          frame #1 {
                            n1188 = Bundle(cluster=w2136, "STATUS"=w2133) -> (w2134:T4)  [unwired: 2 in]
                            n1189 = local write "RESULT LAB05-2"(TRUE) -> ()
                            n1190 = local write "DISP LAB05-2"(w2134) -> ()
                          }
                        }
                      }
                      frame False {
                      }
                    }
                  }
                }
              }
            }
          }
          frame #5 {
            # "check if test cycles reached for temperature rise test"
            n1191 = stacked-sequence {
              tunnel: w2166 -> [_ _ _ _ _ _ _ _ _ _]
              tunnel: w2165 -> [_ _ _ _ _ _ _ _ _ _]
              tunnel: w2164 -> [_ _ _ _ _ _ _ _ _ _]
              tunnel: w2163 -> [_ _ _ _ _ _ _ _ _ _]
              tunnel: w2162 -> [_ _ _ _ _ _ _ _ _ _]
              tunnel: w2161 -> [_ _ _ _ _ _ _ _ _ _]
              tunnel: w2160 -> [_ _ _ _ _ _ _ _ _ _]
              tunnel: w2159 -> [_ _ _ _ _ _ _ _ _ _]
              tunnel: w2158 -> [_ _ _ _ _ _ _ _ _ _]
              tunnel: w2157 -> [_ _ _ _ _ _ _ _ _ _]
              tunnel: w2156 -> [w2172 _ _ _ _ _ _ _ _ _]
              tunnel: w2146 -> [w2167 _ _ _ _ _ _ _ _ _]
              tunnel: w2155 -> [_ w2198 _ _ _ _ _ _ _ _]
              tunnel: w2154 -> [_ _ w2228 _ _ _ _ _ _ _]
              tunnel: w2153 -> [_ _ _ w2258 _ _ _ _ _ _]
              tunnel: w2152 -> [_ _ _ _ w2288 _ _ _ _ _]
              tunnel: w2151 -> [_ _ _ _ _ w2318 _ _ _ _]
              tunnel: w2150 -> [_ _ _ _ _ _ w2348 _ _ _]
              tunnel: w2149 -> [_ _ _ _ _ _ _ w2378 _ _]
              tunnel: w2148 -> [_ _ _ _ _ _ _ _ w2408 _]
              tunnel: w2147 -> [_ _ _ _ _ _ _ _ _ w2438]
              tunnel: w2145 -> [_ w2197 _ _ _ _ _ _ _ _]
              tunnel: w2144 -> [_ _ w2227 _ _ _ _ _ _ _]
              tunnel: w2143 -> [_ _ _ w2257 _ _ _ _ _ _]
              tunnel: w2142 -> [_ _ _ _ w2287 _ _ _ _ _]
              tunnel: w2141 -> [_ _ _ _ _ w2317 _ _ _ _]
              tunnel: w2140 -> [_ _ _ _ _ _ w2347 _ _ _]
              tunnel: w2139 -> [_ _ _ _ _ _ _ w2377 _ _]
              tunnel: w2138 -> [_ _ _ _ _ _ _ _ w2407 _]
              tunnel: w2137 -> [_ _ _ _ _ _ _ _ _ w2437]
              frame #0 {
                # "LAB01-1"
                n1192 = Equal?(x=w2172, y=2) -> (x = y?=w2170:bool)
                n1193 = local read "DISP LAB01-1"() -> (w2173:T4)
                n1194 = Unbundle(w2173) -> ("STATUS"=w2174:string)  [unwired: 2 out]
                n1195 = Equal?(x=w2174, y="RUN") -> (x = y?=w2169:bool)
                n1196 = And(x=w2169, y=w2170) -> (x .and. y?=w2168:bool)
